vi "close.vi"(8 "error in (no error)":errorcluster, 11 "SpinCore in":refnum<class "SpinCore.lvclass">) -> (0 "error out":errorcluster)   [LabVIEW 2011, in "Hardware.lvlib" / "Channels.lvlib" / "SpinCore.lvclass"]
uses:
  SpinCore.lvclass
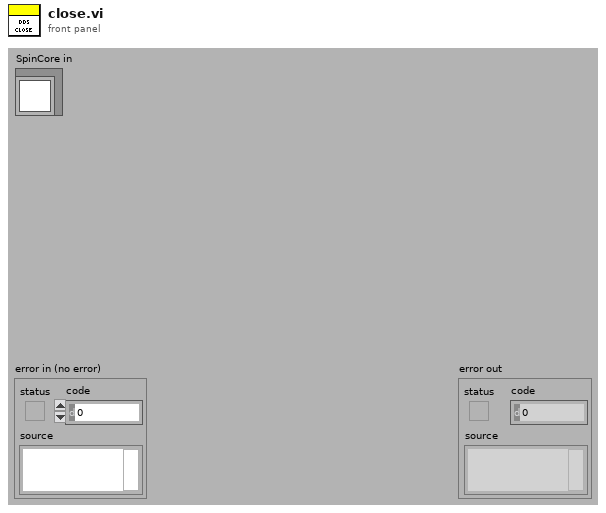
[diagram p1: front panel]
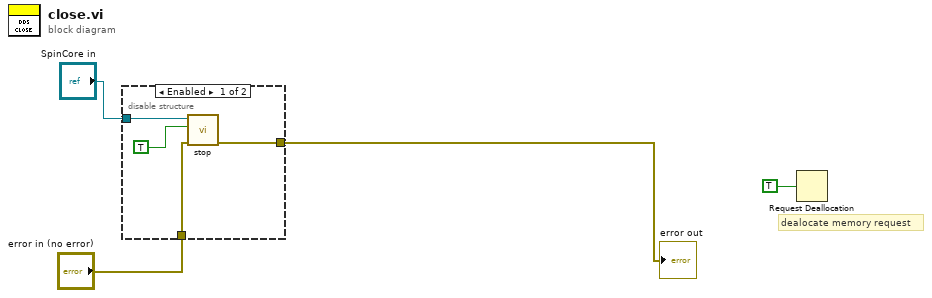
[diagram p0: block diagram]
diagram:
  # "dealocate memory request"
  n1 = disable-structure shown="Enabled" {
    disable-tunnel: "SpinCore in" -> [w8 _]
    disable-tunnel: "error in (no error)" -> [w7 w9]
    disable-tunnel: [w5 w9] -> w1
    frame Enabled {
      n2 = call-dynamic "stop.vi"("error in (no error)"=w7, "stop?"=TRUE, "SpinCore in"=w8) -> ("error out"=w5:errorcluster)  [unwired: 6 in, 2 out]
    }
    frame Disabled {
    }
  }
  "error out" <- w1
  n3 = Request Deallocation(TRUE ("flag")) -> ()
